vi "player_new.vi"() -> ()   [LabVIEW 2010]
uses:
  player_glo.vi
  musicplayer_glo.vi
panel:
  out "playState":i32(ring) items=["wmppsUndefined", "wmppsStopped", "wmppsPaused", "wmppsPlaying", "wmppsScanForward", "wmppsScanReverse", "wmppsBuffering", "wmppsWaiting", "wmppsMediaEnded", "wmppsTransitioning", "wmppsReady", "wmppsReconnecting", "wmppsLast"]
  in  "started?":bool
  in  "WindowsMediaPlayer":refnum<k7>(container)
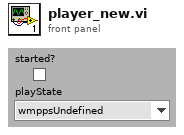
[diagram p1: front panel]
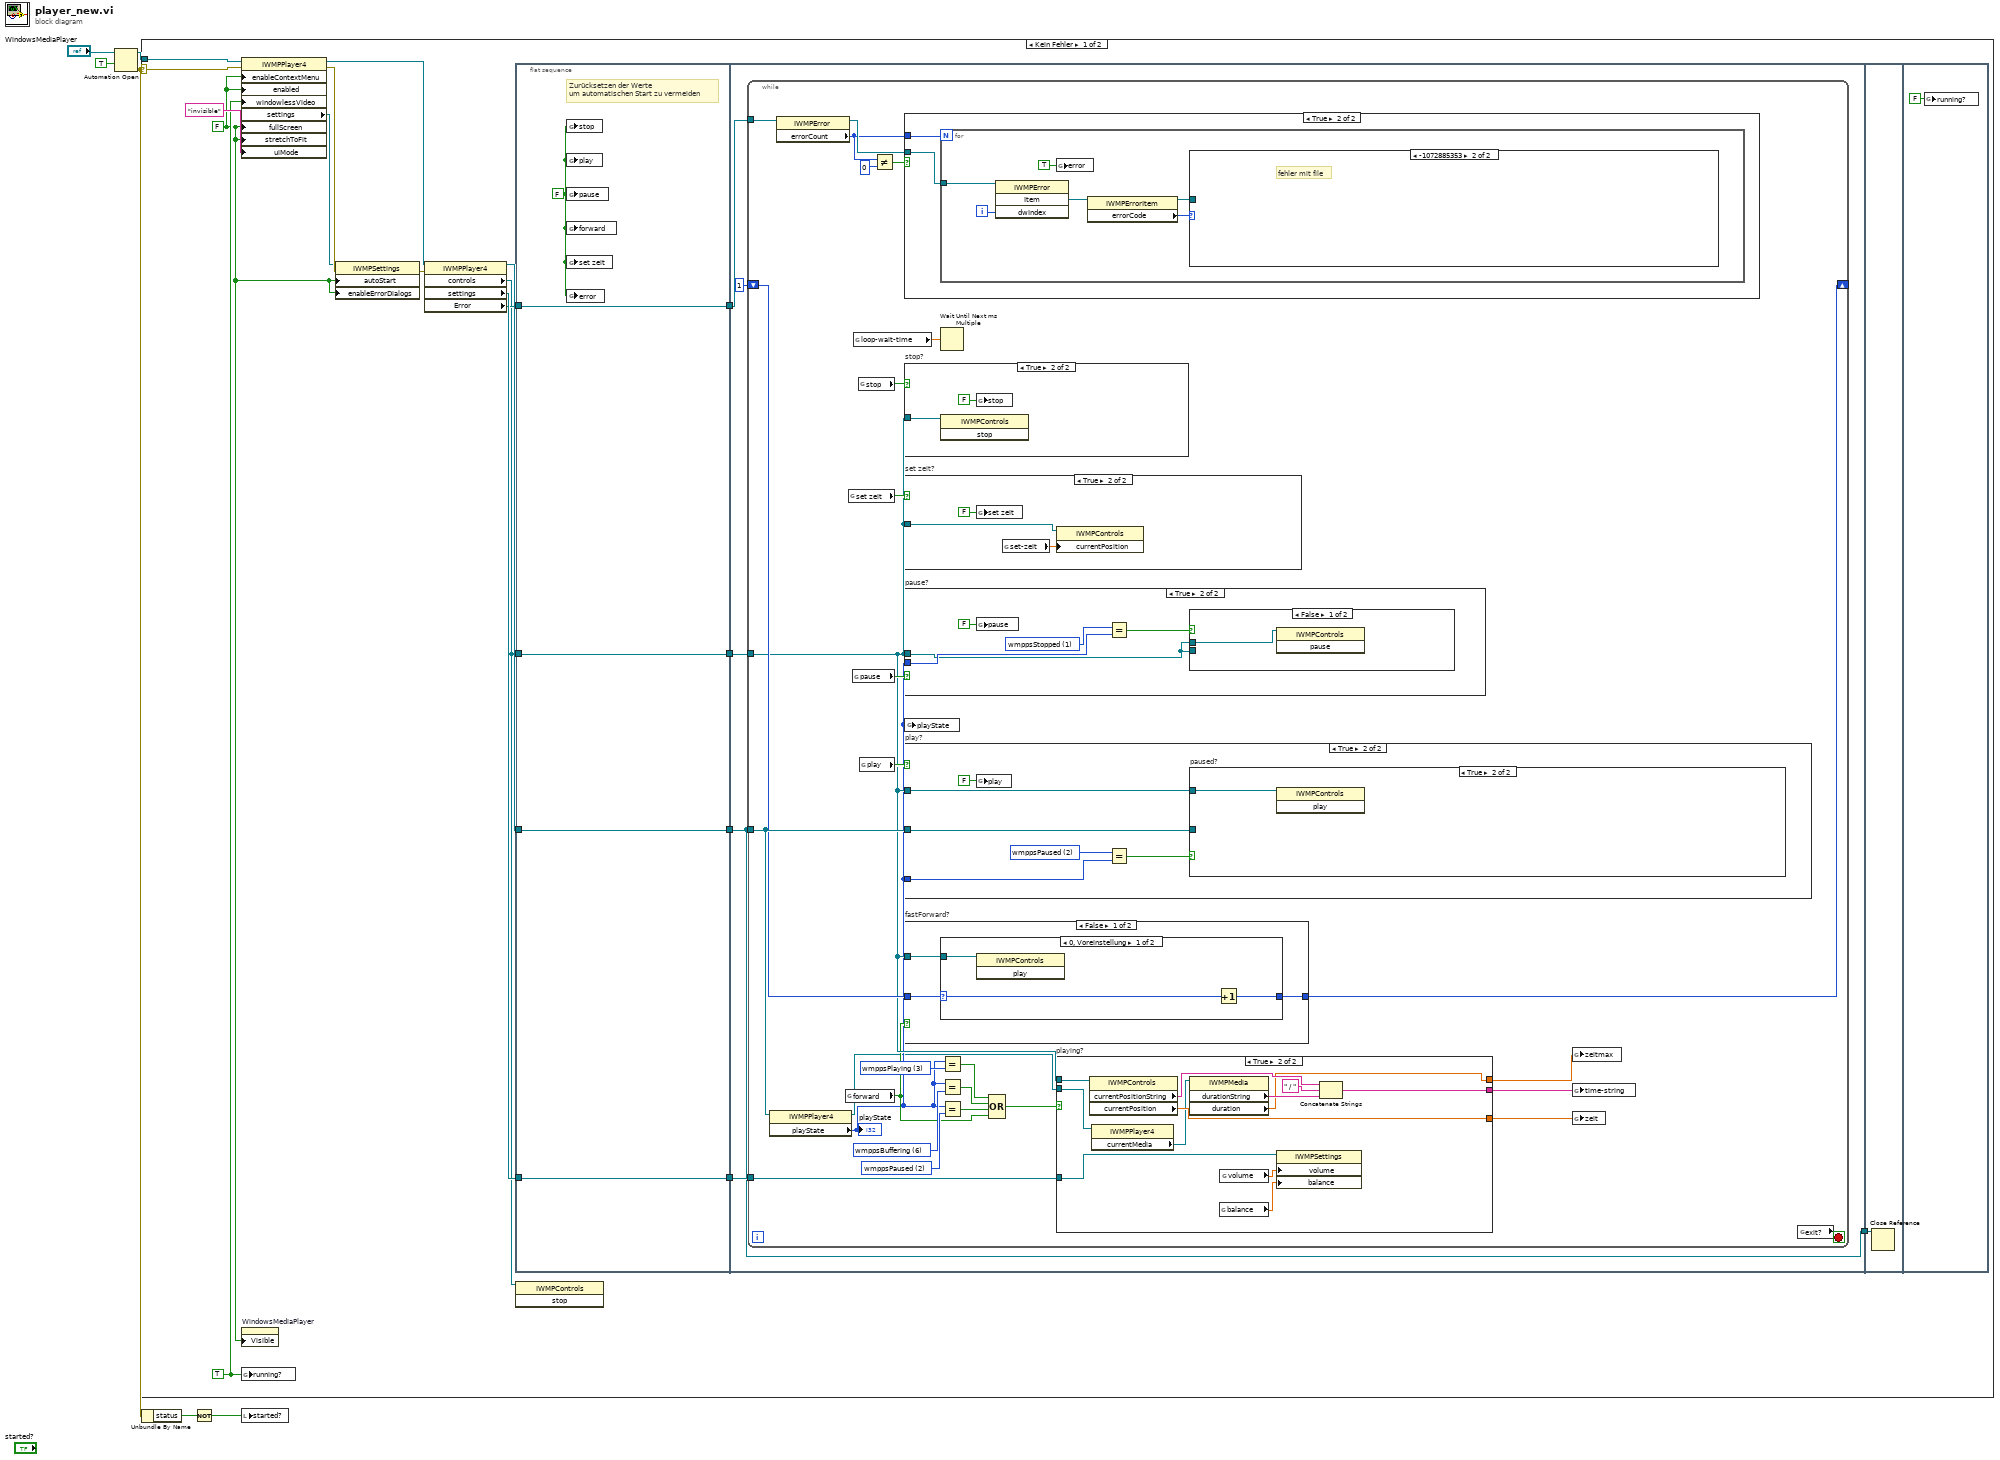
[diagram p0: block diagram]
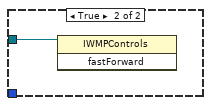
[diagram p3: hidden frame]
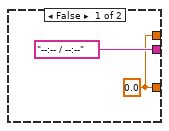
[diagram p5: hidden frame]
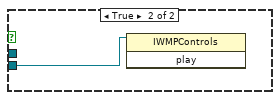
[diagram p7: hidden frame]
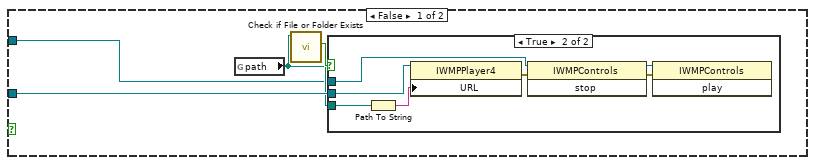
[diagram p10: hidden frame]
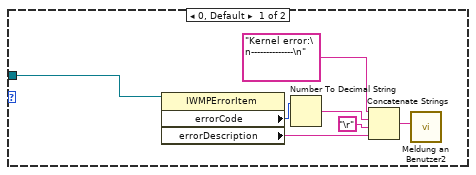
[diagram p13: hidden frame]
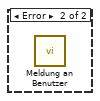
[diagram p14: hidden frame]
diagram:
  n1 = Automation Open(Automation Refnum="WindowsMediaPlayer", 9:TRUE ("Neue Instanz öffnen (False)")) -> (Automation Refnum=w6:refnum<k7>, error out=w3:errorcluster)  [unwired: 2 in]
  n2 = case shown="Kein Fehler" w3 {
    selector: w3 -> [w19 _]
    tunnel: w6 -> [w20 _]
    frame No Error {
      w13 = TRUE ("windowlessVideo")
      w12 = FALSE ("enableContextMenu")
      n3 = property class="IWMPPlayer4"(reference=w20, error in=w19, "enableContextMenu"=w12, "enabled"=w12, "windowlessVideo"=w13, "fullScreen"=w12, "stretchToFit"=w12, "uiMode"="invisible") -> (reference out=w22:refnum<k7>, error out=w23:errorcluster, "settings"=w21:refnum<k7>)
      n4 = property on="WindowsMediaPlayer" class="AXCont"("Visible"=w12) -> ()  [unwired: 2 in, 2 out]
      n5 = global write "player_glo.vi" "running?"(w13) -> ()
      n6 = property class="IWMPSettings"(reference=w21, error in=w23, "autoStart"=w12, "enableErrorDialogs"=w12) -> (error out=w24:errorcluster)  [unwired: 1 out]
      n7 = property class="IWMPPlayer4"(reference=w22, error in=w24) -> (reference out=w18:refnum<k7>, "controls"=w11:refnum<k7>, "settings"=w17:refnum<k7>, "Error"=w16:refnum<k7>)  [unwired: 1 out]
      n8 = flat-sequence {
        tunnel: w16 -> [w26]
        tunnel: w17 -> [w27]
        tunnel: w11 -> [w28]
        tunnel: w18 -> [w29]
        tunnel: [w29] -> w10
        tunnel: [w28] -> w9
        tunnel: [w27] -> w8
        tunnel: [w26] -> w7
        tunnel: [w31] -> w15
        tunnel: w10 -> [w31]
        tunnel: w9 -> [w34]
        tunnel: w8 -> [w33]
        tunnel: w7 -> [w32]
        tunnel: w15 -> [w131]
        frame #0 {
          w25 = FALSE
          # "Zurücksetzen der Werte\num automatischen Start zu vermeiden"
          n9 = global write "player_glo.vi" "stop"(w25) -> ()
          n10 = global write "player_glo.vi" "play"(w25) -> ()
          n11 = global write "player_glo.vi" "pause"(w25) -> ()
          n12 = global write "player_glo.vi" "forward"(w25) -> ()
          n13 = global write "player_glo.vi" "set zeit"(w25) -> ()
          n14 = global write "player_glo.vi" "error"(w25) -> ()
        }
        frame #1 {
          n15 = while {
            tunnel: w31 -> [w56]
            tunnel: w34 -> [w38]
            tunnel: w33 -> [w48]
            tunnel: w32 -> [w63]
            shift-right: [w39] -> _
            shift-left: 1 -> [w40]
            stop <- w58 stop-if-true
            w46 = 2 items=["wmppsUndefined", "wmppsStopped", "wmppsPaused", "wmppsPlaying", "wmppsScanForward", "wmppsScanReverse", "wmppsBuffering", "wmppsWaiting", "wmppsMediaEnded", "wmppsTransitioning", "wmppsReady", "wmppsReconnecting", "wmppsLast"] ("playState")
            w49 = 6 items=["wmppsUndefined", "wmppsStopped", "wmppsPaused", "wmppsPlaying", "wmppsScanForward", "wmppsScanReverse", "wmppsBuffering", "wmppsWaiting", "wmppsMediaEnded", "wmppsTransitioning", "wmppsReady", "wmppsReconnecting", "wmppsLast"] ("playState")
            w53 = 3 items=["wmppsUndefined", "wmppsStopped", "wmppsPaused", "wmppsPlaying", "wmppsScanForward", "wmppsScanReverse", "wmppsBuffering", "wmppsWaiting", "wmppsMediaEnded", "wmppsTransitioning", "wmppsReady", "wmppsReconnecting", "wmppsLast"] ("playState")
            n16 = property class="IWMPPlayer4"(reference=w56) -> (reference out=w35:refnum<k7>, "playState"=w36:i32)  [unwired: 1 in, 1 out]
            "playState" <- w36
            n17 = property class="IWMPError"(reference=w63) -> (reference out=w61:refnum<k7>, "errorCount"=w59:i32)  [unwired: 1 in, 1 out]
            n18 = global read "player_glo.vi" "forward"() -> (w37:bool)
            n19 = global read "player_glo.vi" "set zeit"() -> (w41:bool)
            n20 = global read "player_glo.vi" "pause"() -> (w54:bool)
            n21 = global read "player_glo.vi" "loop-wait-time"() -> (w47:dbl)
            n22 = global read "player_glo.vi" "stop"() -> (w55:bool)
            n23 = global read "player_glo.vi" "play"() -> (w57:bool)
            n24 = Not Equal?(x=w59, y=0) -> (x != y?=w62:bool)
            n25 = case shown="True" w62 {
              tunnel: w61 -> [_ w117]
              tunnel: w59 -> [_ w116]
              frame False {
              }
              frame True {
                n26 = for {
                  N: w116 -> [_]
                  tunnel: w117 -> [w123]
                  i -> [w122]
                  n27 = invoke class="IWMPError" method="Item"(reference=w123, "dwIndex"=w122) -> ("Item"=w121:refnum<k7>)  [unwired: 2 in, 3 out]
                  n28 = global write "player_glo.vi" "error"(TRUE ("error")) -> ()
                  n29 = property class="IWMPErrorItem"(reference=w121) -> (reference out=w119:refnum<k7>, "errorCode"=w120:i32)  [unwired: 1 in, 1 out]
                  n30 = case shown="-1072885353" w120 {
                    tunnel: w119 -> [w128 _]
                    frame 0, Default {
                      n31 = property class="IWMPErrorItem"(reference=w128) -> ("errorCode"=w127:i32, "errorDescription"=w124:string)  [unwired: 1 in, 2 out]
                      n32 = Number To Decimal String(number=w127) -> (decimal integer string=w126:string)  [unwired: 1 in]
                      n33 = Concatenate Strings("Kernel error:\n--------------\n" ("String"), w126, "\r", w124) -> (w130:string)
                      n34 = call "Meldung an Benutzer2"("Message"=w130) -> ()  [unwired: 9 in, 2 out]
                    }
                    frame -1072885353 {
                      # "fehler mit file"
                    }
                  }
                }
              }
            }
            n35 = case "stop?" shown="True" w55 {
              tunnel: w38 -> [_ w96]
              frame False {
              }
              frame True {
                n36 = invoke class="IWMPControls" method="stop"(reference=w96) -> ()  [unwired: 2 in, 3 out]
                n37 = global write "player_glo.vi" "stop"(FALSE) -> ()
              }
            }
            n38 = case "set zeit?" shown="True" w41 {
              tunnel: w38 -> [_ w74]
              frame False {
              }
              frame True {
                n39 = global write "player_glo.vi" "set zeit"(FALSE) -> ()
                n40 = global read "player_glo.vi" "set-zeit"() -> (w73:dbl)
                n41 = property class="IWMPControls"(reference=w74, "currentPosition"=w73) -> ()  [unwired: 1 in, 2 out]
              }
            }
            n42 = case "pause?" shown="True" w54 {
              tunnel: w38 -> [_ w89]
              tunnel: w36 -> [_ w91]
              frame False {
              }
              frame True {
                w92 = 1 items=["wmppsUndefined", "wmppsStopped", "wmppsPaused", "wmppsPlaying", "wmppsScanForward", "wmppsScanReverse", "wmppsBuffering", "wmppsWaiting", "wmppsMediaEnded", "wmppsTransitioning", "wmppsReady", "wmppsReconnecting", "wmppsLast"] ("playState")
                n43 = global write "player_glo.vi" "pause"(FALSE ("pause")) -> ()
                n44 = Equal?(x=w92, y=w91) -> (x = y?=w90:bool)
                n45 = case shown="False" w90 {
                  tunnel: w89 -> [_ w95]
                  tunnel: w89 -> [w94 _]
                  frame False {
                    n46 = invoke class="IWMPControls" method="pause"(reference=w94) -> ()  [unwired: 2 in, 3 out]
                  }
                  frame True {
                    n47 = invoke class="IWMPControls" method="play"(reference=w95) -> ()  [unwired: 2 in, 3 out]
                  }
                }
              }
            }
            n48 = global write "player_glo.vi" "playState"(w36) -> ()
            n49 = case "play?" shown="True" w57 {
              tunnel: w38 -> [_ w102]
              tunnel: w56 -> [_ w103]
              tunnel: w36 -> [_ w99]
              frame False {
              }
              frame True {
                w101 = 2 items=["wmppsUndefined", "wmppsStopped", "wmppsPaused", "wmppsPlaying", "wmppsScanForward", "wmppsScanReverse", "wmppsBuffering", "wmppsWaiting", "wmppsMediaEnded", "wmppsTransitioning", "wmppsReady", "wmppsReconnecting", "wmppsLast"] ("playState")
                n50 = global write "player_glo.vi" "play"(FALSE ("play")) -> ()
                n51 = Equal?(x=w101, y=w99) -> (x = y?=w100:bool)
                n52 = case "paused?" shown="True" w100 {
                  tunnel: w103 -> [w106 _]
                  tunnel: w102 -> [w104 w115]
                  frame False {
                    n53 = global read "player_glo.vi" "path"() -> (w105:path)
                    n54 = call <vilib>:"Check if File or Folder Exists.vi"("path"=w105) -> ("file or folder exists?"=w107:bool)  [unwired: 8 in, 2 out]
                    n55 = case shown="True" w107 {
                      tunnel: w106 -> [_ w112]
                      tunnel: w105 -> [_ w114]
                      tunnel: w104 -> [_ w110]
                      frame False {
                      }
                      frame True {
                        n56 = Path To String(path=w114) -> (string=w113:string)
                        n57 = property class="IWMPPlayer4"(reference=w112, "URL"=w113) -> (error out=w111:errorcluster)  [unwired: 1 in, 1 out]
                        n58 = invoke class="IWMPControls" method="stop"(reference=w110, error in=w111) -> (reference out=w109:refnum<k7>, error out=w108:errorcluster)  [unwired: 1 in, 1 out]
                        n59 = invoke class="IWMPControls" method="play"(reference=w109, error in=w108) -> ()  [unwired: 1 in, 3 out]
                      }
                    }
                  }
                  frame True {
                    n60 = invoke class="IWMPControls" method="play"(reference=w115) -> ()  [unwired: 2 in, 3 out]
                  }
                }
              }
            }
            n61 = case "fastForward?" shown="False" w37 {
              tunnel: w38 -> [w66 w71]
              tunnel: w40 -> [w65 _]
              tunnel: [w64 _] -> w39
              frame False {
                n62 = case shown="0, Voreinstellung" w65 {
                  selector: w65 -> [w69 w70]
                  tunnel: w66 -> [w67 _]
                  tunnel: [w68 w70] -> w64
                  frame 0, Default {
                    n63 = invoke class="IWMPControls" method="play"(reference=w67) -> ()  [unwired: 2 in, 3 out]
                    n64 = Increment(x=w69) -> (x+1=w68:i32)
                  }
                  frame 1 {
                  }
                }
              }
              frame True {
                n65 = invoke class="IWMPControls" method="fastForward"(reference=w71) -> ()  [unwired: 2 in, 3 out]
              }
            }
            n66 = Wait Until Next ms Multiple(millisecond multiple=w47) -> ()  [unwired: 1 out]
            n67 = Equal?(x=w36, y=w53) -> (x = y?=w52:bool)
            n68 = Equal?(x=w36, y=w49) -> (x = y?=w50:bool)
            n69 = Equal?(x=w36, y=w46) -> (x = y?=w45:bool)
            n70 = Compound Arithmetic op=OR(w52, w50, w45, w37) -> (w51:bool)
            n71 = case "playing?" shown="True" w51 {
              tunnel: w48 -> [_ w86]
              tunnel: w38 -> [_ w85]
              tunnel: ["--:-- / --:--" w81] -> w44
              tunnel: [w75 w80] -> w43
              tunnel: [w75 w79] -> w42
              tunnel: w35 -> [_ w78]
              frame False {
                w75 = 0.0 ("currentPosition")
              }
              frame True {
                n72 = property class="IWMPControls"(reference=w85) -> ("currentPositionString"=w84:string, "currentPosition"=w80:dbl)  [unwired: 1 in, 2 out]
                n73 = property class="IWMPPlayer4"(reference=w78) -> ("currentMedia"=w77:refnum<k7>)  [unwired: 1 in, 2 out]
                n74 = property class="IWMPMedia"(reference=w77) -> ("durationString"=w82:string, "duration"=w79:dbl)  [unwired: 1 in, 2 out]
                n75 = global read "player_glo.vi" "balance"() -> (w88:dbl)
                n76 = global read "player_glo.vi" "volume"() -> (w87:dbl)
                n77 = property class="IWMPSettings"(reference=w86, "volume"=w87, "balance"=w88) -> ()  [unwired: 1 in, 2 out]
                n78 = Concatenate Strings(w84, " / ", w82) -> (w81:string)
              }
            }
            n79 = global write "player_glo.vi" "zeitmax"(w42) -> ()
            n80 = global write "player_glo.vi" "time-string"(w44) -> ()
            n81 = global write "player_glo.vi" "zeit"(w43) -> ()
            n82 = global read "musicplayer_glo.vi" "exit?"() -> (w58:bool)
          }
        }
        frame #2 {
          n83 = Close Reference(reference=w131) -> ()  [unwired: 1 in, 1 out]
        }
        frame #3 {
          n84 = global write "player_glo.vi" "running?"(FALSE) -> ()
        }
      }
      n85 = invoke class="IWMPControls" method="stop"(reference=w11) -> ()  [unwired: 2 in, 3 out]
    }
    frame Error {
      n86 = call "Meldung an Benutzer"() -> ()  [unwired: 3 in, 9 out]
    }
  }
  n87 = Unbundle By Name(w3) -> ("status"=w2:bool)
  n88 = Not(x=w2) -> (.not. x?=w1:bool)
  n89 = local write "started?"(w1) -> ()
